vi "Outputs.vi"(8 "error in (no error)":errorcluster, 11 "State in":T1={"State"=enum."Idle", "Start Time"=timestamp(0 s since 1904-01-01), "Current Time"=timestamp(0 s since 1904-01-01), "First Iteration"=FALSE, "Process Name"="", "Output Error"=FALSE, "Log Started"=FALSE, "Cycle Period"=0.0, "Configuration"={"Valve Settings"={"D-O Settings"={"DAQmx Task Name"="", "Output Channel"=0, "Output Channel Names"=[]}, "VICI Electronic Actuator"={"VISA resource name"="", "Mode"=enum."Two Positions With Stops", "Simulated"=FALSE}}, "Valve Type"=enum."Digital Output Valve", "Time On (Sec)"=0.0, "Time Off (Sec)"=0.0, "Run?"=FALSE}, "Data"={"D-O State"=enum."Off"}} {"Configuration"."Valve Settings"."D-O Settings"."Output Channel" items=["Choose a Channel"]}) -> (0 "error out":errorcluster, 3 "State out":T1={"State"=enum."Idle", "Start Time"=timestamp(0 s since 1904-01-01), "Current Time"=timestamp(0 s since 1904-01-01), "First Iteration"=FALSE, "Process Name"="", "Output Error"=FALSE, "Log Started"=FALSE, "Cycle Period"=50.0, "Configuration"={"Valve Settings"={"D-O Settings"={"DAQmx Task Name"="", "Output Channel"=0, "Output Channel Names"=[]}, "VICI Electronic Actuator"={"VISA resource name"="", "Mode"=enum."Two Positions With Stops", "Simulated"=FALSE}}, "Valve Type"=enum."Default", "Time On (Sec)"=0.0, "Time Off (Sec)"=0.0, "Run?"=FALSE}, "Data"={"D-O State"=enum."Off"}} {"Configuration"."Valve Settings"."D-O Settings"."Output Channel" items=["Choose a Channel"]})   [LabVIEW 2018]
uses:
  State Cluster.ctl
  State Enum.ctl
  Valve Clusters.ctl
  D-O Module Settings Cluster.ctl
  D-O Device Settings Cluster.ctl
  VICI Electronic Actuator/VICI Electronic Actuator Settings.ctl
  Tag VIs/Tag FGV Operation Enum.ctl
  <vilib>/DAQmx/write.llb/DAQmx Write (Digital Bool 1Line 1Point).vi
  <vilib>/DAQmx/miscellaneous.llb/DAQmx Fill In Error Info.vi
  D-O Module Engine.lvlib
  Shared Variables/Dynamic Shared Variables.lvlib
  D-O Module.lvlib
  DIO Valve/VICI Electronic Actuator.lvlib
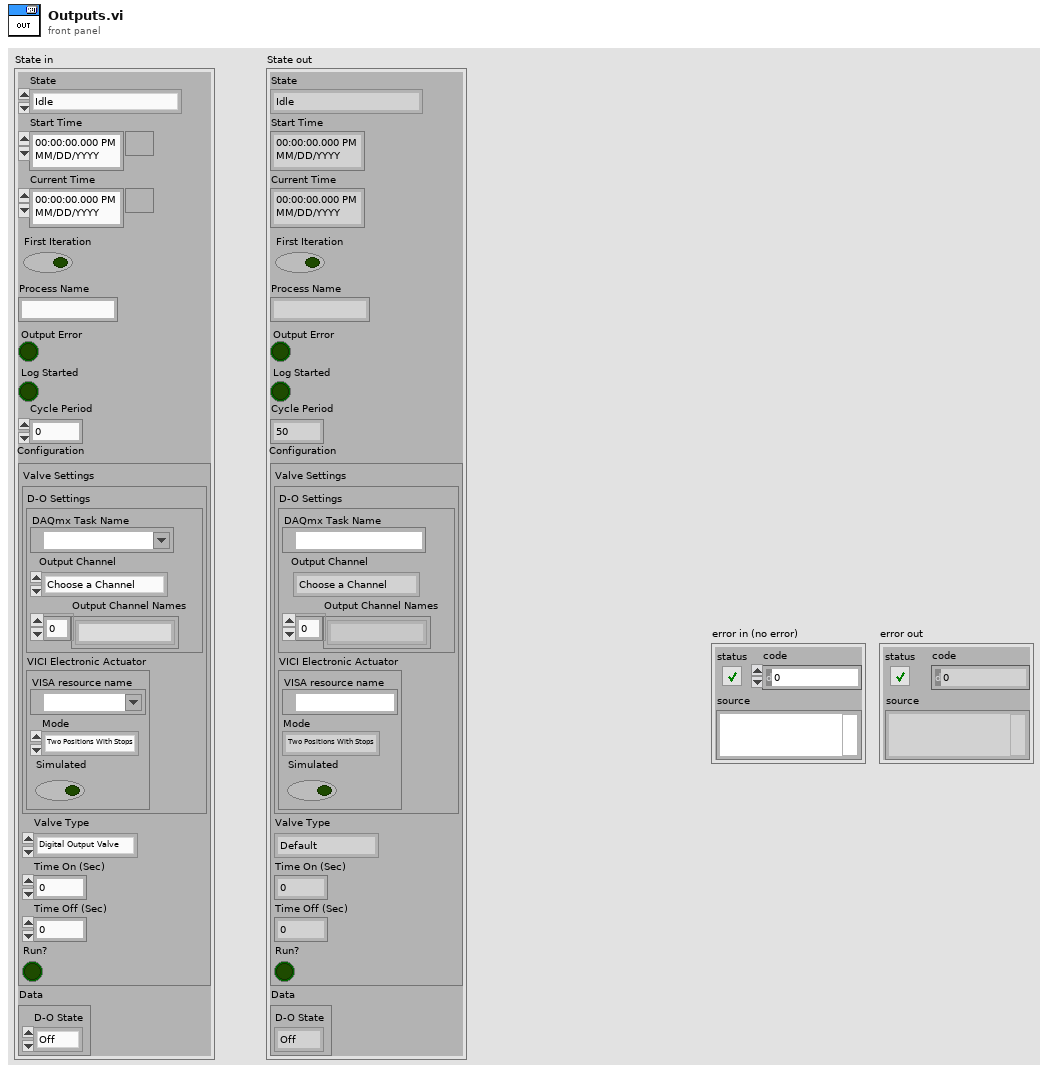
[diagram p1: front panel]
types:
  T1 = typedef "D-O Module.lvlib/D-O Module Engine.lvlib/State Cluster.ctl" = cluster{"State":T2, "Start Time":timestamp, "Current Time":timestamp, "First Iteration":bool, "Process Name":string, "Output Error":bool, "Log Started":bool, "Cycle Period":dbl, "Configuration":T3, "Data":cluster{"D-O State":enum16{"Off", "On", "Not Initialized"}}}
  T2 = typedef "D-O Module.lvlib/D-O Module Engine.lvlib/State Enum.ctl" = enum16{"Measuring", "Idle", "Paused"}
  T3 = typedef "D-O Module.lvlib/Valve Clusters.ctl" = cluster{"Valve Settings":T4, "Valve Type":enum16{"Default", "Digital Output Valve", "VICI Electronic Actuator"}, "Time On (Sec)":dbl, "Time Off (Sec)":dbl, "Run?":bool}
  T4 = typedef "D-O Module.lvlib/D-O Module Settings Cluster.ctl" = cluster{"D-O Settings":T5, "VICI Electronic Actuator":T6}
  T5 = typedef "D-O Module.lvlib/D-O Device Settings Cluster.ctl" = cluster{"DAQmx Task Name":refnum<k21>, "Output Channel":u16, "Output Channel Names":string[]}
  T6 = typedef "VICI Electronic Actuator.lvlib/VICI Electronic Actuator Settings.ctl" = cluster{"VISA resource name":refnum<visa-resource-name>, "Mode":enum16{"Two Positions With Stops", "Two Positions Without Stops", "Mutiposition"}, "Simulated":bool}
  T7 = typedef "Tag FGV Operation Enum.ctl" = enum16{"Init", "Set Notification Queue", "Create Tag", "Commit", "Write Tag (Numeric)", "Write Tag (Boolean)", "Read All Tags", "Read One Tag", "Delete Tag Category", "Set Alarm Parameters (Numeric)", "Set Alarm Parameters (Boolean)", "Enable All Alarms", "Disable All Alarms", "Delete All Tags", "Read Alarms", "Ack Alarm", "Read Alarm Parameters (Numeric)", "Read Alarm Parameters (Boolean)"}
  T8 = typedef "D-O Module.lvlib/D-O Module Tag Names Cluster.ctl" = cluster{"D-O Status":string, "Identifier Tag":string}
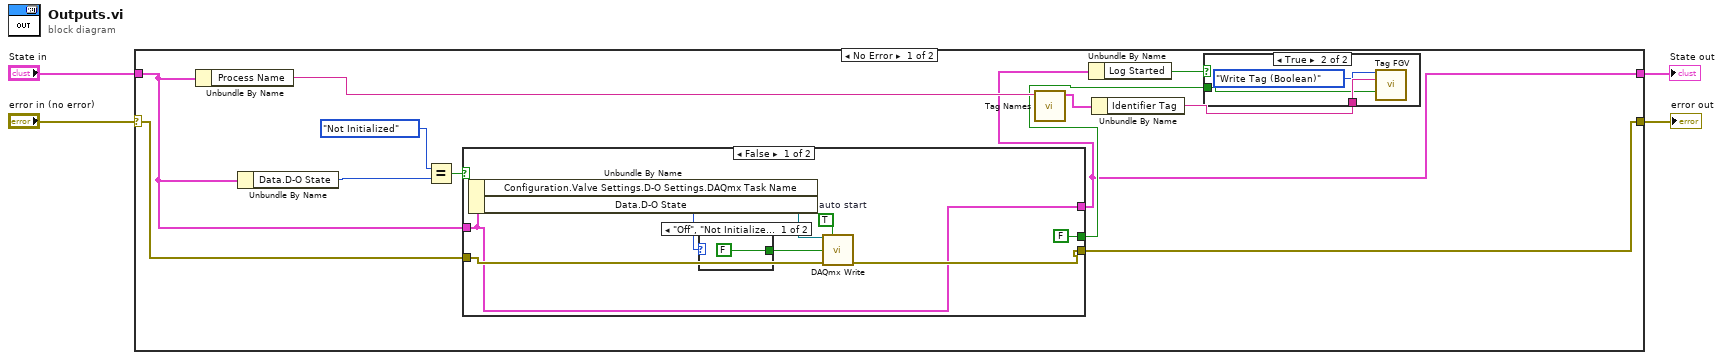
[diagram p0: block diagram]
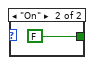
[diagram p3: hidden frame]
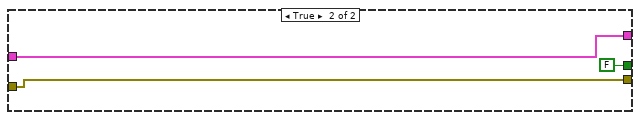
[diagram p4: hidden frame]
diagram:
  n1 = case shown="No Error" "error in (no error)" {
    selector: "error in (no error)" -> [w16 w34]
    tunnel: [w13 w34] -> w3
    tunnel: "State in" -> [w12 w33]
    tunnel: [w6 w33] -> w1
    frame No Error {
      n2 = Unbundle By Name(w12) -> ("Process Name"=w15:string)
      n3 = Unbundle By Name(w12) -> ("Data.D-O State"=w9:enum16{"Off", "On", "Not Initialized"})
      n4 = Equal?(x=enum16{"Off", "On", "Not Initialized"}."Not Initialized", y=w9) -> (x = y?=w7:bool)
      n5 = case shown="False" w7 {
        tunnel: w16 -> [w23 w30]
        tunnel: [w21 w31] -> w6
        tunnel: [w22 w30] -> w13
        tunnel: w12 -> [w21 w31]
        tunnel: [FALSE ("Connection Error") FALSE ("Connection Error")] -> w10
        frame False {
          w26 = TRUE  # auto start
          n6 = Unbundle By Name(w21) -> ("Configuration.Valve Settings.D-O Settings.DAQmx Task Name"=w25:refnum<k21>, "Data.D-O State"=w27:enum16{"Off", "On", "Not Initialized"})
          n7 = case shown="\"Off\", \"Not Initialized\", Default" w27 {
            tunnel: [FALSE ("D-O State") FALSE ("D-O State")] -> w24
            frame "Off", "Not Initialized", Default {
            }
            frame "On" {
            }
          }
          n8 = call-poly <vilib>:"DAQmx Write.vi"("task/channels in"=w25, "auto start"=w26, "data"=w24, "error in"=w23) -> ("error out"=w22:errorcluster)  [unwired: 9 in, 2 out]
        }
        frame True {
        }
      }
      n9 = call "Tag Names.vi"("Process Name"=w15) -> ("Pump Module Tag Names"=w14:T8)  [unwired: 8 in, 2 out]
      n10 = Unbundle By Name(w6) -> ("Log Started"=w5:bool)
      n11 = Unbundle By Name(w14) -> ("Identifier Tag"=w11:string)
      n12 = case shown="True" w5 {
        tunnel: w11 -> [_ w19]
        tunnel: w10 -> [_ w18]
        frame False {
        }
        frame True {
          n13 = call "Tag FGV.vi"("Operation"=Tag_FGV_Operation_Enum."Write Tag (Boolean)", "Tag Name"=w19, "Data"=w18) -> ()  [unwired: 5 in, 8 out]
        }
      }
    }
    frame Error {
    }
  }
  "error out" <- w3
  "State out" <- w1
